vi "WriteChannelAliasName.vi"(8 "error in (no error)":errorcluster, 10 "ChannelAliasName":string, 11 "DataVer2 in":refnum<class "DataVer2.lvclass">) -> (0 "error out":errorcluster, 3 "DataVer2 out":refnum<class "DataVer2.lvclass">)   [LabVIEW 2013, in "DataVer2.lvclass"]
uses:
  DataVer2.lvclass
  DataVer2.lvclass/DataVer2.ctl
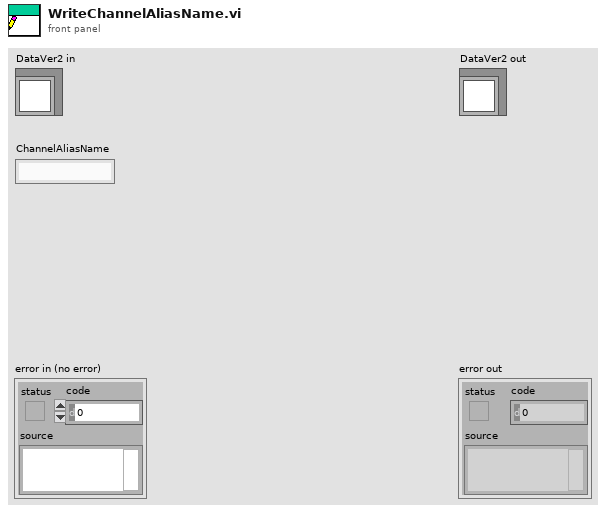
[diagram p1: front panel]
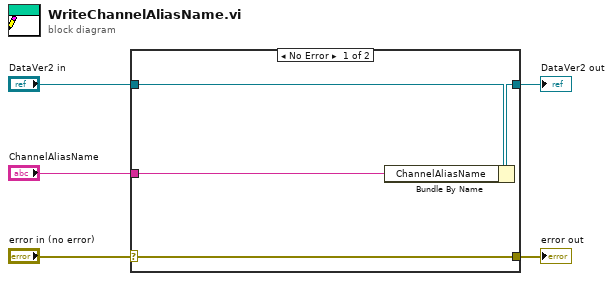
[diagram p0: block diagram]
diagram:
  n1 = case shown="No Error" "error in (no error)" {
    selector: "error in (no error)" -> [w9 w10]
    tunnel: [w9 w10] -> w4
    tunnel: [w7 w11] -> w2
    tunnel: "DataVer2 in" -> [w8 w11]
    tunnel: "ChannelAliasName" -> [w6 _]
    frame No Error {
      n2 = Bundle By Name(cluster=w8, "ChannelAliasName"=w6) -> (w7:refnum<class "DataVer2.lvclass">)
    }
    frame Error {
    }
  }
  "error out" <- w4
  "DataVer2 out" <- w2
